vi "Read NumScans.vi"(8 "error in (no error)":errorcluster, 11 "SEDSpectrometer in":refnum<class "SEDSpectrometer.lvclass">) -> (0 "error out":errorcluster, 2 "NumScans":i16=-1 caption="Nr Of Scans", 3 "SEDSpectrometer out":refnum<class "SEDSpectrometer.lvclass">)   [LabVIEW 2016, in "SEDSpectrometer.lvclass"]
uses:
  SEDSpectrometer.lvclass
  SEDSpectrometer.lvclass/SEDSpectrometer.ctl
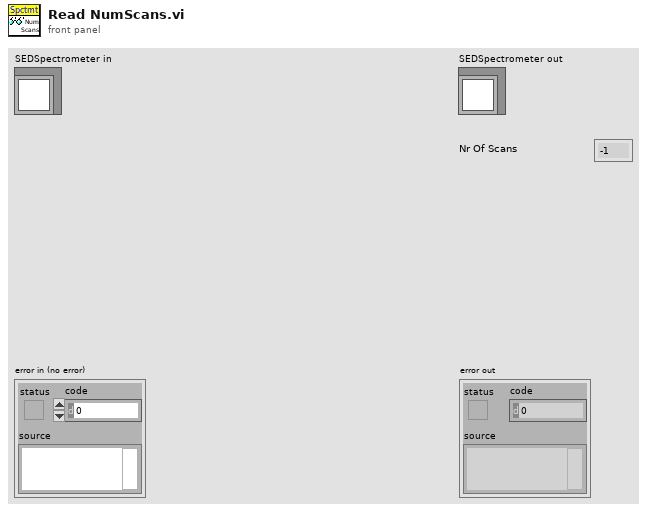
[diagram p1: front panel]
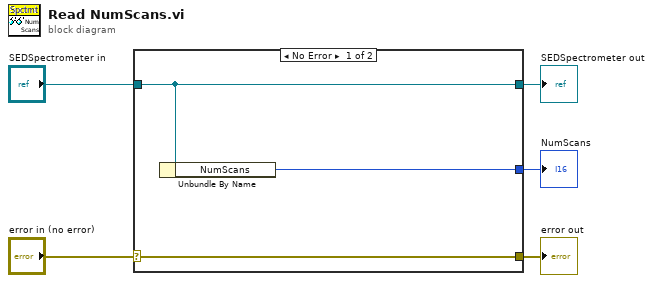
[diagram p0: block diagram]
diagram:
  n1 = case shown="No Error" "error in (no error)" {
    selector: "error in (no error)" -> [w8 w9]
    tunnel: [w8 w9] -> w4
    tunnel: [w7 w10] -> w2
    tunnel: "SEDSpectrometer in" -> [w7 w10]
    tunnel: [w6 _] -> w1
    frame No Error {
      n2 = Unbundle By Name(w7) -> ("NumScans"=w6:i16)
    }
    frame Error {
    }
  }
  "error out" <- w4
  "SEDSpectrometer out" <- w2
  "NumScans" <- w1
